vi "Check and Reestablish Connection.vi"(9 "CD Path":string, 10 "IP Address":string, 11 "connection info":T1) -> (0 "error out":errorcluster, 3 "connection info":T1)   [LabVIEW 2023, in "J1939 Workspace Shared.lvlib"]
uses:
  J1939 Workspace Shared.lvlib
  <vilib>/NI/STM/TCP/TCP Connection Info.ctl
  <vilib>/NI/STM/SubVIs/MetaDataElement.ctl
  Addon/Addon Shared/J1939 Addon Shared.lvlib
  <vilib>/NI/STM/NI STM.lvlib
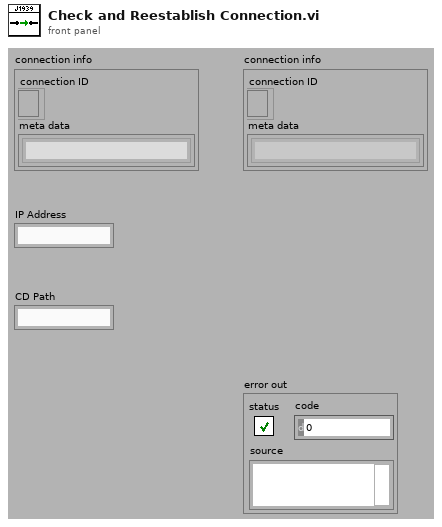
[diagram p1: front panel]
types:
  T1 = typedef "NI STM.lvlib/TCP Connection Info.ctl" = cluster{"connection ID":refnum<k5>, "meta data":T2[]}
  T2 = typedef "NI STM.lvlib/MetaDataElement.ctl" = string
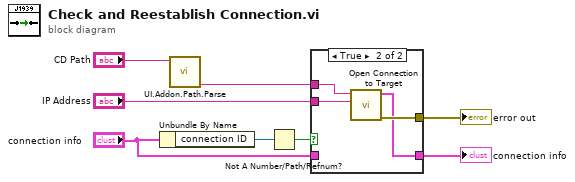
[diagram p0: block diagram]
diagram:
  n1 = Unbundle By Name("connection info") -> ("connection ID"=w3:refnum<k5>)
  n2 = call "UI.Addon.Path.Parse.vi"("Cached Addon Path"="CD Path") -> ("Addon Name"=w1:string)  [unwired: 6 in, 4 out]
  n3 = Not A Number/Path/Refnum?(number/path/refnum=w3) -> (NaN/Path/Refnum?=w7:bool)
  n4 = case shown="True" w7 {
    tunnel: w1 -> [_ w11]
    tunnel: [w9 w12] -> w5
    tunnel: "connection info" -> [w9 _]
    tunnel: [_ w13] -> w8
    tunnel: "IP Address" -> [_ w10]
    frame False {
    }
    frame True {
      n5 = call "Open Connection to Target.vi"("IP Address"=w10, "TCP Service"=w11) -> ("error out"=w13:errorcluster, "connection info"=w12:T1)  [unwired: 8 in]
    }
  }
  "error out" <- w8
  "connection info" <- w5
